vi "Add Team.vi"(8 "error in (no error)":errorcluster, 10 "Team Type":refnum<class "Team.lvclass">, 11 "Game in":refnum<class "Game.lvclass">) -> (0 "error out":errorcluster, 2 "Team":refnum<class "Team.lvclass">, 3 "Game out":refnum<class "Game.lvclass">)   [LabVIEW 2020, in "SquareBattle.lvlib" / "Game.lvclass"]
uses:
  Game.lvclass
  Team/Team.lvclass
  Game.lvclass/Game.ctl
  Team ID.ctl
  Team/Team.lvclass/Team.ctl
  <vilib>/Utility/miscctls.llb/LVMapReplaceAction.ctl
  Map/Map.lvclass
  SquareBattle.lvlib
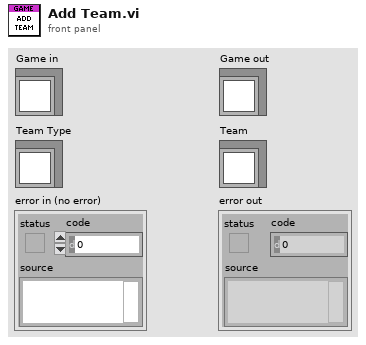
[diagram p1: front panel]
types:
  T1 = typedef "SquareBattle.lvlib/Team ID.ctl" = u32
  T2 = typedef "LVMapReplaceAction.ctl" = enum32{"Modify Entry only if found", "Add or Modify Entry", "Delete Entry"}
  T3 = typedef "SquareBattle.lvlib/Position.ctl" = cluster{"Row":i32, "Col":i32}
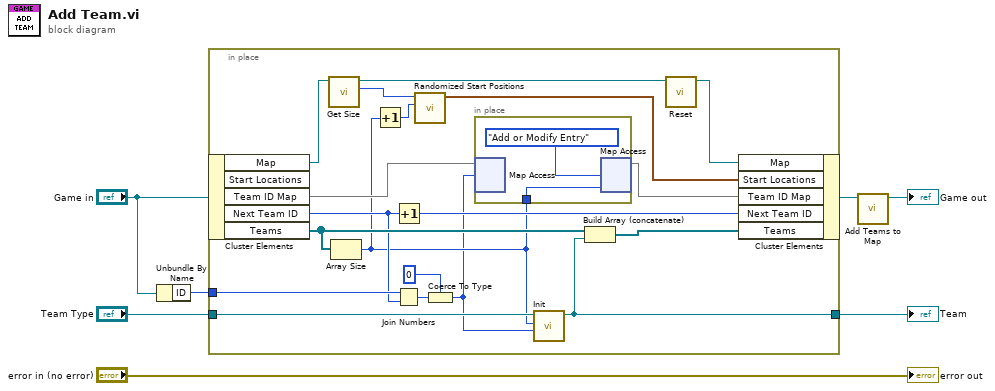
[diagram p0: block diagram]
diagram:
  n1 = Unbundle By Name("Game in") -> ("ID"=w4:u16)
  n2 = in-place {
    in-place-border: "Team Type" -> [w26]
    in-place-border: [w24] -> w5
    in-place-border: w4 -> [w21]
    n3 = in-place-cluster #1("Game in") -> ("Map"=w12:refnum<class "Map.lvclass">, "Team ID Map"=w19:map{T1, i32}, "Next Team ID"=w20:u16, "Teams"=w25:refnum<class "Team.lvclass">[])  [unwired: 1 out]
    n4 = call "Get Size.vi"("Map in"=w12) -> ("Size"=w14:i32, "Map out"=w11:refnum<class "Map.lvclass">)  [unwired: 9 in]
    n5 = Array Size(array=w25) -> (size(s)=w16:i32)
    n6 = Increment(x=w16) -> (x+1=w15:i32)
    n7 = Increment(x=w20) -> (x+1=w22:u16)
    n8 = Join Numbers(hi=w21, lo=w20) -> ((hi.lo)=w18:u32)
    n9 = call "Randomized Start Positions.vi"("Player Count"=w15, "Size"=w14) -> ("Positions"=w13:T3[])  [unwired: 9 in]
    n10 = Coerce To Type(0:w18, 1:T1 0 ("Team ID")) -> (2:w8:T1)
    n11 = in-place {
      in-place-border: w16 -> [w27]
      n12 = in-place-map #2(w19, w8) -> ()  [unwired: 1 in, 2 out]
      n13 = in-place-map #2(w27, LVMapReplaceAction."Add or Modify Entry" ("action")) -> (w17:map{T1, i32})  [unwired: 2 out]
    }
    n14 = call "Init.vi"("Team ID"=w8, "Index"=w16, "Team in"=w26) -> ("Team out"=w24:refnum<class "Team.lvclass">)  [unwired: 8 in]
    n15 = Build Array (concatenate)(w25, w24) -> (w23:refnum<class "Team.lvclass">[])
    n16 = call "Reset.vi"("Map in"=w11) -> ("Map out"=w10:refnum<class "Map.lvclass">)  [unwired: 9 in, 1 out]
    n17 = in-place-cluster #1("Map"=w10, "Start Locations"=w13, "Team ID Map"=w17, "Next Team ID"=w22, "Teams"=w23) -> (w2:refnum<class "Game.lvclass">)
  }
  "Team" <- w5
  n18 = call "Add Teams to Map.vi"("Game in"=w2) -> ("Game out"=→"Game out":refnum<class "Game.lvclass">)  [unwired: 10 in]
  "error out" <- "error in (no error)"
